vi "gRPC Server.vi"(8 "error in (no error)":errorcluster, 11 "CIFTemplatePlugin in":refnum<class "Template_Plugin.lvclass">) -> (0 "error out":errorcluster, 3 "CIFTemplatePlugin out":refnum<class "Template_Plugin.lvclass">)   [LabVIEW 2021, in "Template_Plugin.lvclass"]
uses:
  Template_Plugin.lvclass
  Template_Plugin.lvclass/Template_Plugin.ctl
  <vilib>/CIF Foundation/CIF Core/CIFCore/Class/CIFCorePlugin.lvclass
  Grpc/Template_server/RPC Service/Template/Template.lvclass
  Grpc/Template_server/RPC Messages/cif_template_Status.ctl
  Grpc/Template_server/Template_server.lvlib
  Grpc/Template_server/RPC Messages/cif_template_Result.ctl
  C:/Program Files/National Instruments/LabVIEW 2021/vi.lib/CIF Foundation/CIF Core/CIFCore/Class/CIFCorePlugin.lvclass
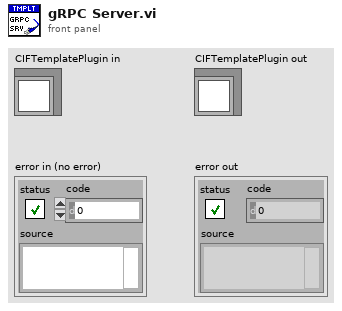
[diagram p1: front panel]
types:
  T1 = typedef "Template_server.lvlib/cif_Template_Status.ctl" = cluster{"code":i32, "message":string}
  T2 = typedef "grpc-lvsupport-release.lvlib/grpcId.ctl" = u64
  T3 = typedef "Template_server.lvlib/cif_Template_Numeric.ctl" = cluster{"numeric":i32}
  T4 = typedef "Template_server.lvlib/cif_Template_Result.ctl" = cluster{"result":i32}
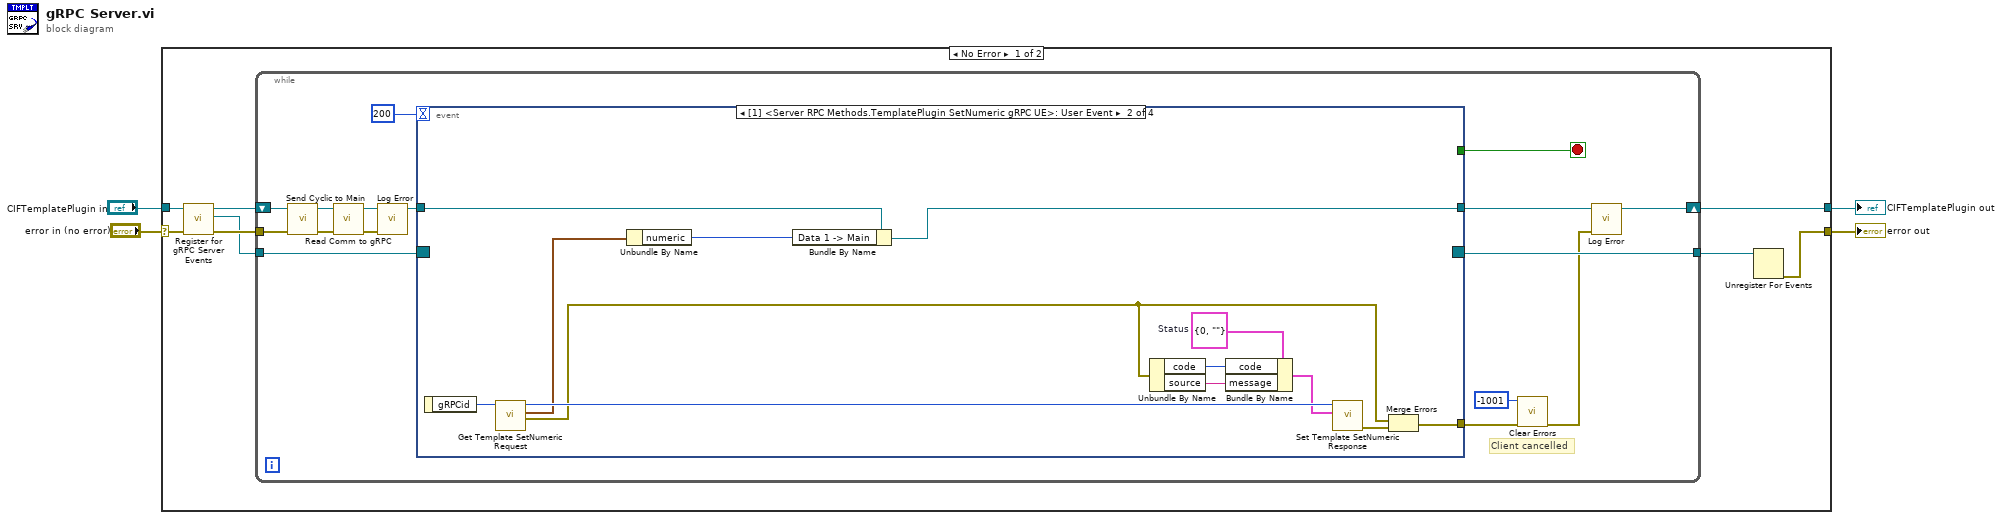
[diagram p0: block diagram]
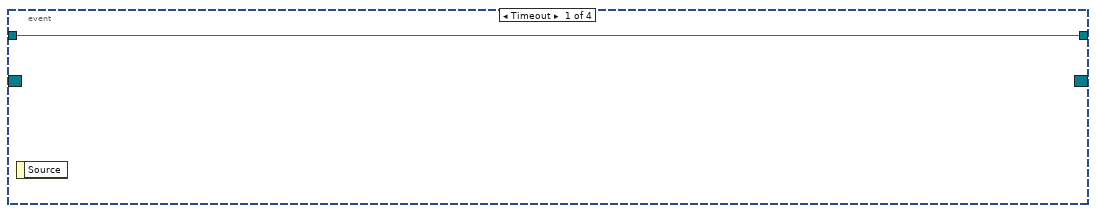
[diagram p2: hidden frame]
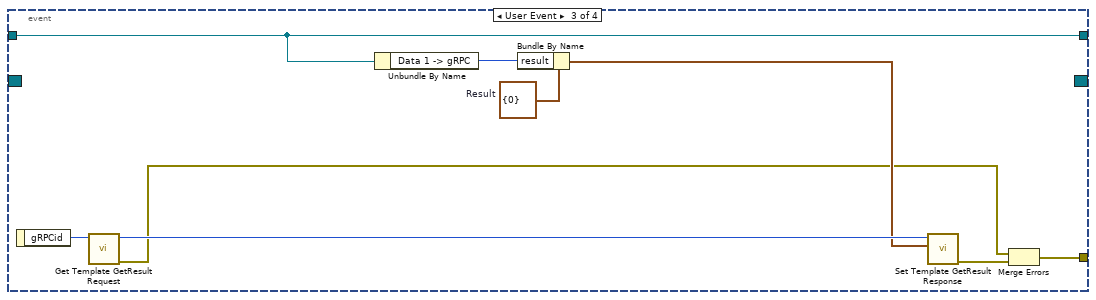
[diagram p3: hidden frame]
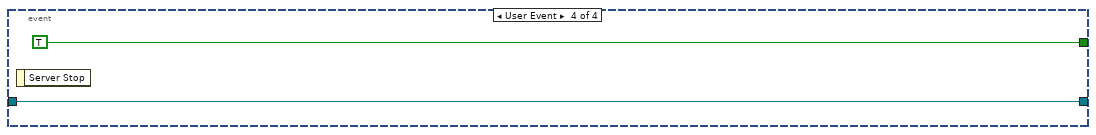
[diagram p4: hidden frame]
diagram:
  n1 = case shown="No Error" "error in (no error)" {
    selector: "error in (no error)" -> [w9 w54]
    tunnel: "CIFTemplatePlugin in" -> [w10 w55]
    tunnel: [w11 w55] -> w3
    tunnel: [w6 w54] -> w4
    frame No Error {
      n2 = call "Register for gRPC Server Events.vi"("error in (no error)"=w9, "CIFTemplatePlugin in"=w10) -> ("error out"=w8:errorcluster, "Event Registration Refnum"=w5:refnum<event-registration>, "CIFTemplatePlugin out"=w7:refnum<class "Template_Plugin.lvclass">)  [unwired: 7 in]
      n3 = while {
        tunnel: w5 -> [w28]
        tunnel: w8 -> [w20]
        tunnel: [w25] -> w12
        shift-right: [w23] -> w11
        shift-left: w7 -> [w21]
        stop <- w26 stop-if-true
        # "Client cancelled"
        n4 = call "Send Cyclic to Main.vi"("error in (no error)"=w20, "CIFTemplatePlugin in"=w21) -> ("error out"=w18:errorcluster, "CIFTemplatePlugin out"=w19:refnum<class "Template_Plugin.lvclass">)  [unwired: 8 in]
        n5 = call "Read Comm to gRPC.vi"("error in (no error)"=w18, "CIFTemplatePlugin in"=w19) -> ("error out"=w16:errorcluster, "CIFTemplatePlugin out"=w17:refnum<class "Template_Plugin.lvclass">)  [unwired: 8 in]
        n6 = call <vilib>:"Log Error.vi"("error in (no error)"=w16, "CIFCorePlugin in"=w17) -> ("CIFCorePlugin in"=w22:refnum<class "Template_Plugin.lvclass">)  [unwired: 8 in, 1 out]
        n7 = event shown="[1] <Server RPC Methods.TemplatePlugin SetNumeric gRPC UE>: User Event" {
          selector: w28 -> [_ _ _ _]
          dyn-events: [_ _ _ _] -> w25
          timeout: 200 -> [_ _ _ _]
          tunnel: w22 -> [w29 w33 w50 w52]
          tunnel: [_ w40 w51 _] -> w14
          tunnel: [w29 w31 w50 w52] -> w24
          tunnel: [_ _ _ TRUE] -> w26
          event Timeout {
            n8 = event-data() -> ()  [unwired: 1 in, 1 out]
          }
          event User Event {
            w35 = T1 {"code"=0, "message"=""}  # Status
            n9 = event-data() -> ("gRPCid"=w38:T2)  [unwired: 1 in]
            n10 = call "Get Template SetNumeric Request.vi"("gRPCid"=w38) -> ("error out"=w30:errorcluster, "Message Data"=w34:T3, "gRPCid out"=w39:T2)  [unwired: 8 in]
            n11 = Unbundle By Name(w34) -> ("numeric"=w32:i32)
            n12 = Bundle By Name(cluster=w33, "Data 1 -> Main"=w32) -> (w31:refnum<class "Template_Plugin.lvclass">)
            n13 = Unbundle By Name(w30) -> ("code"=w42:i32, "source"=w41:string)
            n14 = Bundle By Name(cluster=w35, "code"=w42, "message"=w41) -> (w37:T1)
            n15 = call "Set Template SetNumeric Response.vi"("Message Data"=w37, "gRPCid in"=w39) -> ("error out"=w36:errorcluster)  [unwired: 9 in]
            n16 = Merge Errors(w30, w36) -> (w40:errorcluster)
          }
          event User Event {
            w45 = T4 {"result"=0}  # Result
            n17 = event-data() -> ("gRPCid"=w48:T2)  [unwired: 1 in]
            n18 = call "Get Template GetResult Request.vi"("gRPCid"=w48) -> ("error out"=w44:errorcluster, "gRPCid out"=w47:T2)  [unwired: 8 in, 1 out]
            n19 = Unbundle By Name(w50) -> ("Data 1 -> gRPC"=w49:i32)
            n20 = Bundle By Name(cluster=w45, "result"=w49) -> (w46:T4)
            n21 = call "Set Template GetResult Response.vi"("Message Data"=w46, "gRPCid in"=w47) -> ("error out"=w43:errorcluster)  [unwired: 9 in]
            n22 = Merge Errors(w44, w43) -> (w51:errorcluster)
          }
          event User Event {
            n23 = event-data() -> ()  [unwired: 1 in, 1 out]
          }
        }
        n24 = call <vilib>:"Clear Errors.vi"("error in (no error)"=w14, "specific error code to clear (0: all)"=-1001) -> ("error out"=w13:errorcluster)  [unwired: 4 in, 1 out]
        n25 = call <vilib>:"Log Error.vi"("error in (no error)"=w13, "CIFCorePlugin in"=w24) -> ("CIFCorePlugin in"=w23:refnum<class "Template_Plugin.lvclass">)  [unwired: 8 in, 1 out]
      }
      n26 = Unregister For Events(event registration refnum=w12) -> (error out=w6:errorcluster)  [unwired: 1 in]
    }
    frame Error {
    }
  }
  "error out" <- w4
  "CIFTemplatePlugin out" <- w3
